vi "Determine Controller.vi"(7 "Processing In":refnum<class "Processing.lvclass">, 11 "Route Handler in":refnum<class "Route Handler.lvclass">) -> (0 "error out":errorcluster, 2 "Controller":refnum<class "Controller.lvclass">, 5 "Processing":refnum<class "Processing.lvclass">)   [LabVIEW 2020, in "HTTP Server.lvlib" / "Route Handler.lvclass"]
uses:
  Route Handler.lvclass
  Processing/Processing.lvclass
  Controller/Controller.lvclass
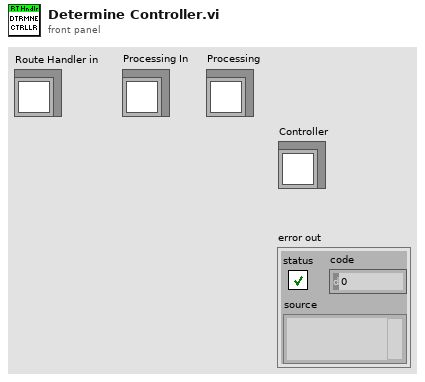
[diagram p1: front panel]
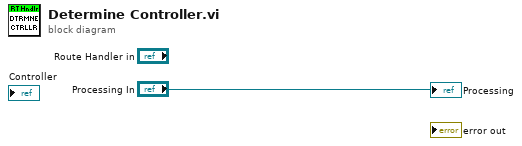
[diagram p0: block diagram]
diagram:
  "Processing" <- "Processing In"
